vi "Calculate Kalman Gain.vi"(9 "R":T1, 10 "H":T1, 11 "Prior Covariance":T1) -> (3 "Kalman Gain":T1)   [LabVIEW 2020]
uses:
  <vilib>/Analysis/Matrix/Datatypes/RealMatrix.ctl
  <vilib>/Analysis/7linalg.llb/Real Transpose Matrix.vi
  <vilib>/Analysis/baseanly.llb/Real A x B.vi
  <vilib>/Analysis/Matrix/Numeric/Add/Add - RM,RM.vi
  <vilib>/Analysis/baseanly.llb/Real Inverse Matrix.vi
  <vilib>/Analysis/NI_AALBase.lvlib
  <vilib>/Analysis/NI_AALPro.lvlib
  <vilib>/Analysis/Matrix/NI_Matrix.lvlib
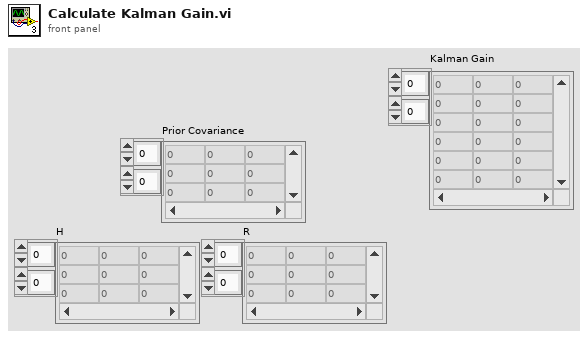
[diagram p1: front panel]
types:
  T1 = typedef "NI_Matrix.lvlib/RealMatrix.ctl" = dbl[][]
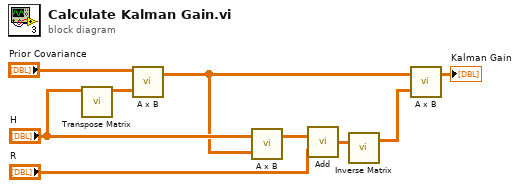
[diagram p0: block diagram]
diagram:
  n1 = call-poly <vilib>:"Transpose Matrix.vi"("Input Matrix"="H") -> ("Matrix Transpose"=w8:T1)  [unwired: 9 in, 1 out]
  n2 = call-poly <vilib>:"A x B.vi"("B"=w8, "A"="Prior Covariance") -> ("A x B"=w1:T1)  [unwired: 1 out]
  n3 = call-poly <vilib>:"A x B.vi"("B"=w1, "A"="H") -> ("A x B"=w7:T1)  [unwired: 1 out]
  n4 = call-poly <vilib>:"Add.vi"("Real Matrix B"="R", "Real Matrix A"=w7) -> ("A + B"=w5:T1)
  n5 = call-poly <vilib>:"Inverse Matrix.vi"("Input Matrix"=w5) -> ("Inverse Matrix"=w4:T1)  [unwired: 1 in, 1 out]
  n6 = call-poly <vilib>:"A x B.vi"("B"=w4, "A"=w1) -> ("A x B"=→"Kalman Gain":T1)  [unwired: 1 out]
